vi "CalculateYaw.vi"(1 "ay":dbl, 2 "ax":dbl) -> (0 "yaw":dbl)   [LabVIEW 2015]
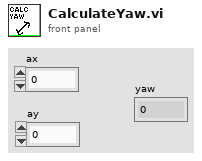
[diagram p1: front panel]
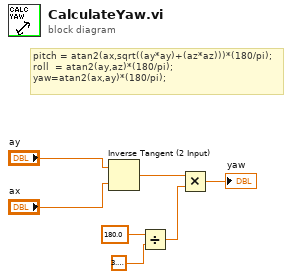
[diagram p0: block diagram]
diagram:
  # "pitch = atan2(ax,sqrt((ay*ay)+(az*az)))*(180/pi);\nroll  = atan2(ay,az)*(180/pi);\nyaw=atan2(ax,ay)*(180/pi);"
  n1 = Inverse Tangent (2 Input)(1:"ax", 2:"ay") -> (0:w7:dbl)
  n2 = Divide(x=180.0, y=3.141592653589793) -> (x/y=w4:dbl)
  n3 = Multiply(x=w7, y=w4) -> (x*y=→"yaw":dbl)
